vi "My Read Lines From File.vi"(0 "file path (dialog if empty)":path, 5 "number of lines (all:-1)":i32=-1, 7 "convert eol? (F)":bool, 9 "number of lines to skip (0)":i32, 11 "error in (no error)":errorcluster, 12 "start of read offset (chars.:0)":i32, 13 "max characters/row  (no limit:0)":i32) -> (4 "new file path (Not A Path if cancelled)":path, 6 "line string":string, 8 "mark after read (chars.)":i32, 10 "EOF?":bool, 15 "error out":errorcluster)   [LabVIEW 2021, in "Files.lvlib"]
doc: "Reads a specified number of lines from a byte stream file beginning at a specified character offset. The VI opens the file before reading from it and closes it afterwards."
uses:
  Files.lvlib
panel:
  in  "prompt":string="Choose file to read."
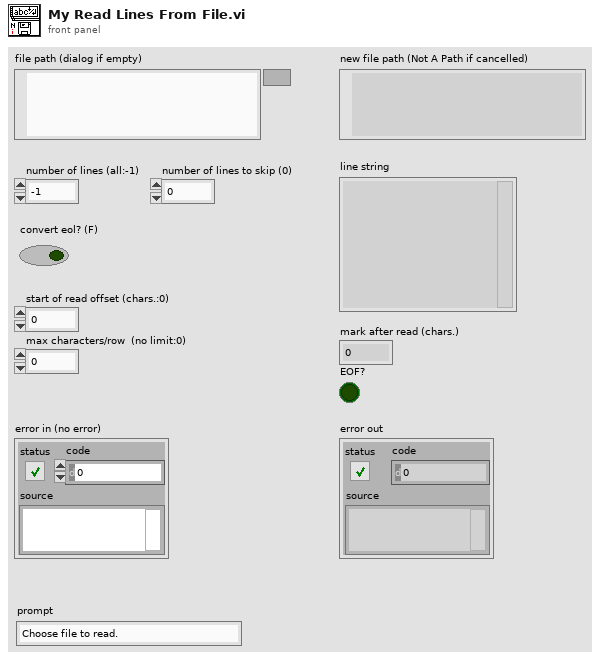
[diagram p1: front panel]
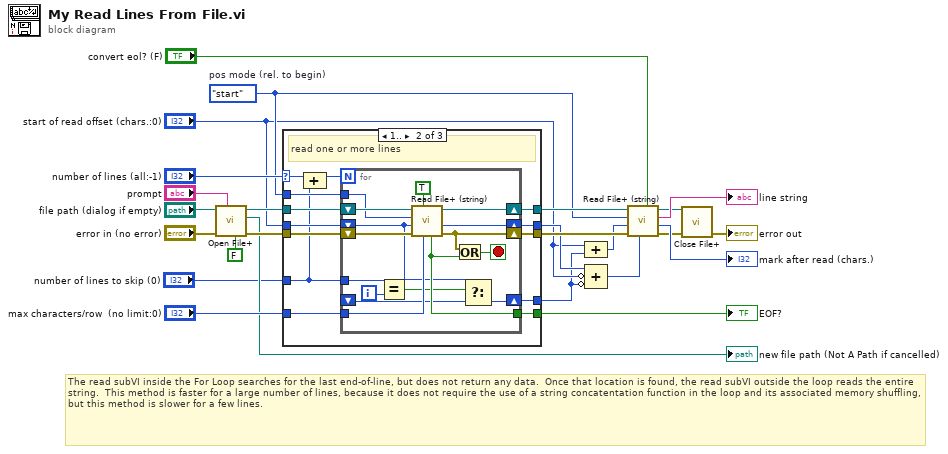
[diagram p0: block diagram]
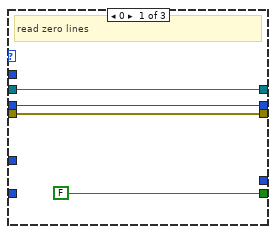
[diagram p2: hidden frame]
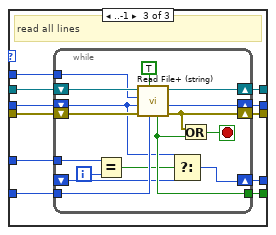
[diagram p3: hidden frame]
diagram:
  w16 = enum16{"start", "end", "current"}."start"  # pos mode (rel. to begin)
  # "The read subVI inside the For Loop searches for the last end-of-line, but does not return any data.  Once that location is found, the read subVI outside the loop reads the entire string.  This method is faster for a large number of lines, because it does not require the use of a string concatentation function in the loop and its associated memory shuffling, but this method is slower for a few lines."
  n1 = call <vilib>:"Open File+.vi"("advisory dialog? (display:T)"=FALSE, "prompt"="prompt", "error in (not an error)"="error in (no error)", "file path (\" \")"="file path (dialog if empty)") -> ("error out"=w15:errorcluster, "file path"=→"new file path (Not A Path if cancelled)":path, "refnum"=w13:refnum<file>)  [unwired: 4 in, 1 out]
  n2 = case shown="1.." "number of lines (all:-1)" {
    selector: "number of lines (all:-1)" -> [_ w33 _]
    tunnel: [w29 w42 w69] -> w22
    tunnel: [w26 w41 w68] -> w21
    tunnel: "max characters/row  (no limit:0)" -> [_ w40 w67]
    tunnel: w15 -> [w29 w39 w66]
    tunnel: w13 -> [w28 w38 w65]
    tunnel: "start of read offset (chars.:0)" -> [w26 w37 w64]
    tunnel: w16 -> [_ w36 w63]
    tunnel: [w28 w35 w62] -> w19
    tunnel: [FALSE w34 w61] -> w18
    tunnel: "number of lines to skip (0)" -> [_ w30 w60]
    tunnel: [_ w32 w59] -> w1
    frame 0 {
      # "read zero lines"
    }
    frame 1.. {
      # "read one or more lines"
      n3 = Compound Arithmetic op=ADD(w33, w30) -> (w31:i32)
      n4 = for {
        N: w31 -> [_]
        tunnel: [w51] -> w34
        tunnel: w36 -> [w53]
        tunnel: w40 -> [w55]
        shift-left: w37 -> [w45]
        shift-right: [w58] -> w41
        shift-right: [w50] -> w42
        shift-left: w39 -> [w54]
        shift-right: [w57] -> w35
        shift-left: w38 -> [w56]
        shift-right: [w46] -> w32
        shift-left: _ -> [w47]
        tunnel: w30 -> [w44]
        i -> [w43]
        stop <- w49 stop-if-true
        n5 = Equal?(x=w44, y=w43) -> (x = y?=w48:bool)
        n6 = call <vilib>:"Read File+ (string).vi"("count"=w55, "line mode (characters:F)"=TRUE ("read line"), "error in (no error)"=w54, "pos offset (bytes:0)"=w45, "pos mode (rel. to current:2)"=w53, "refnum"=w56) -> ("error out"=w50:errorcluster, "mark after read (bytes)"=w58:i32, "dup refnum"=w57:refnum<file>, "EOF?"=w51:bool)  [unwired: 1 in, 1 out]
        n7 = Or(x=w50, y=w51) -> (x .or. y?=w49:bool)
        n8 = Select(t=w45, s=w48, f=w47) -> (s? t:f=w46:i32)
      }
    }
    frame ..-1 {
      # "read all lines"
      n9 = while {
        tunnel: [w78] -> w61
        tunnel: w63 -> [w80]
        tunnel: w67 -> [w82]
        shift-left: w64 -> [w73]
        shift-right: [w85] -> w68
        shift-right: [w77] -> w69
        shift-left: w66 -> [w81]
        shift-right: [w84] -> w62
        shift-left: w65 -> [w83]
        shift-right: [w74] -> w59
        shift-left: _ -> [w75]
        tunnel: w60 -> [w71]
        i -> [w70]
        stop <- w72 stop-if-true
        n10 = Equal?(x=w71, y=w70) -> (x = y?=w76:bool)
        n11 = call <vilib>:"Read File+ (string).vi"("count"=w82, "line mode (characters:F)"=TRUE ("read line"), "error in (no error)"=w81, "pos offset (bytes:0)"=w73, "pos mode (rel. to current:2)"=w80, "refnum"=w83) -> ("error out"=w77:errorcluster, "mark after read (bytes)"=w85:i32, "dup refnum"=w84:refnum<file>, "EOF?"=w78:bool)  [unwired: 1 in, 1 out]
        n12 = Select(t=w73, s=w76, f=w75) -> (s? t:f=w74:i32)
        n13 = Or(x=w77, y=w78) -> (x .or. y?=w72:bool)
      }
    }
  }
  "EOF?" <- w18
  n14 = Compound Arithmetic op=ADD("start of read offset (chars.:0)", w1) -> (w3:i32)
  n15 = Compound Arithmetic op=ADD(w21, invert "start of read offset (chars.:0)", invert w1) -> (w25:i32)
  n16 = call <vilib>:"Read File+ (string).vi"("convert eol? (no:F)"="convert eol? (F)", "count"=w25, "error in (no error)"=w22, "pos offset (bytes:0)"=w3, "pos mode (rel. to current:2)"=w16, "refnum"=w19) -> ("error out"=w10:errorcluster, "mark after read (bytes)"=→"mark after read (chars.)":i32, "string"=→"line string":string, "dup refnum"=w8:refnum<file>)  [unwired: 1 in, 1 out]
  n17 = call <vilib>:"Close File+.vi"("error in (no error)"=w10, "refnum"=w8) -> ("error out"=→"error out":errorcluster)  [unwired: 3 in, 2 out]
